vi "Add Correction.vi"(8 "error in (no error)":errorcluster, 9 "Assembly Type":string, 10 "XYZTheta":dbl[](array[numeric]), 11 "Carrier Tray in":refnum<class "Assembly Tray.lvclass">) -> (0 "error out":errorcluster, 2 "XYZTheta Out":dbl[](array[numeric]), 3 "Carrier Tray out":refnum<class "Assembly Tray.lvclass">)   [LabVIEW 2021, in "Assembly Tray.lvclass"]
uses:
  Assembly Tray.lvclass
  C:/Users/HEP/Documents/GitHub/Gantry/UCSB-Gantry-HEP-main/Classes/Workspace/Fixture.lvclass
  Fixture.lvclass/Fixture.ctl
  Read Fixture ID.vi
  Read Position.vi
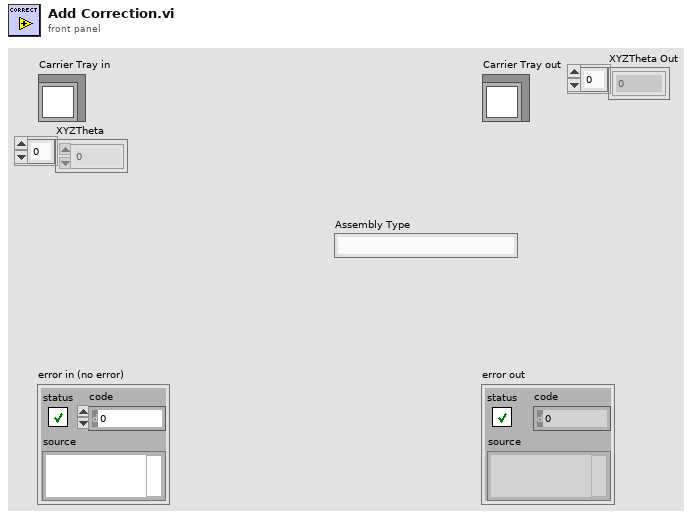
[diagram p1: front panel]
types:
  T1 = typedef "File Paths.ctl" = cluster{"Glue Pattern Folder":path, "Carrier Tray Folder":path, "Pick Up Tool Fixture Folder":path, "Components Folder":path, "Bellows Tool Offset.txt":path, "Pick Up Tool Offset.txt":path, "Dispense Tip Offset.txt":path, "Log Files":path, "Gantry Assembly Map.txt":path, "Syringe and offset map.txt":path, "Controllers Folder":path, "Local dbase config":path}
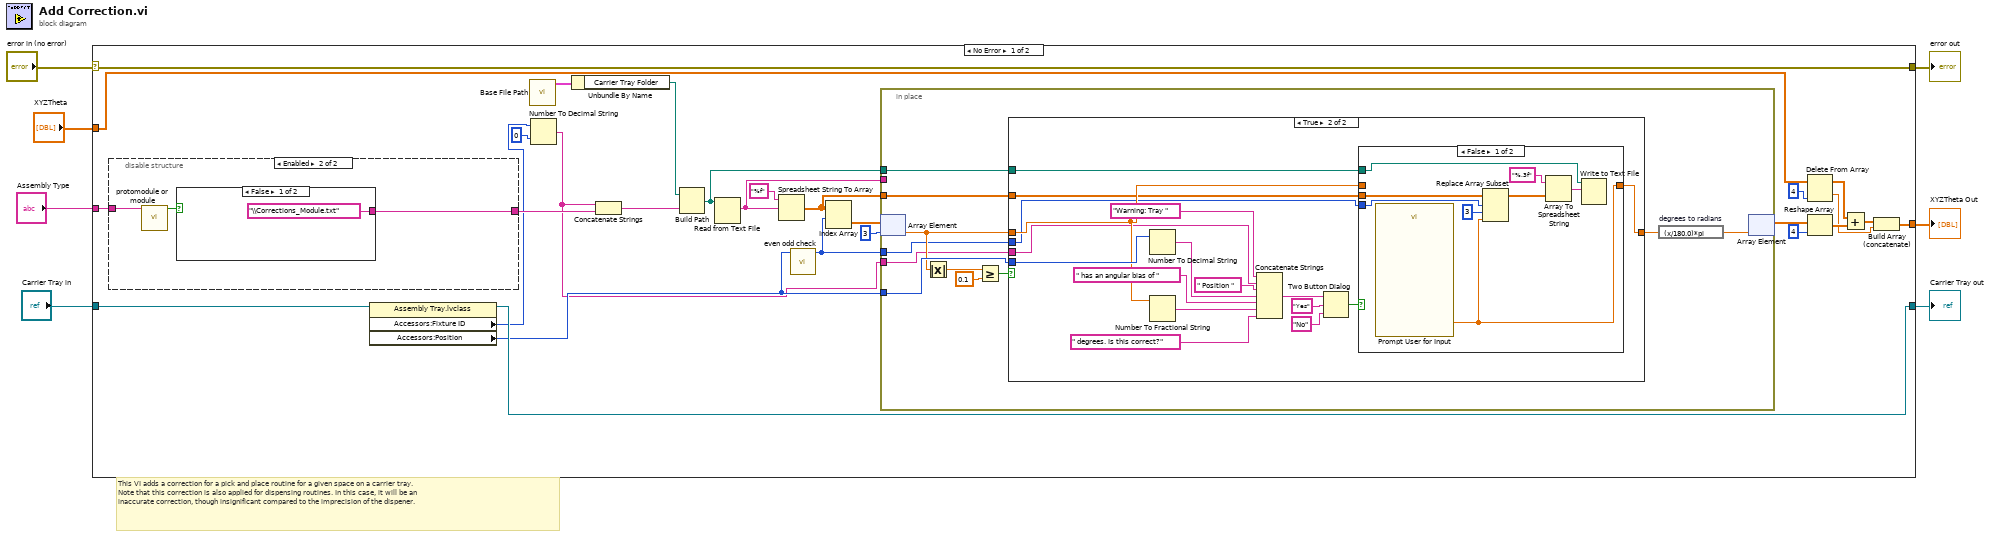
[diagram p0: block diagram]
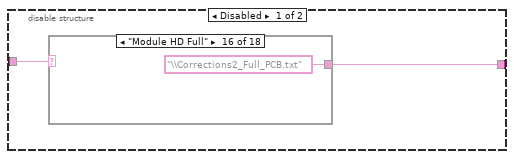
[diagram p4: hidden frame]
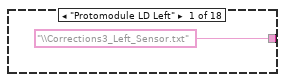
[diagram p5: hidden frame]
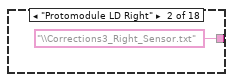
[diagram p6: hidden frame]
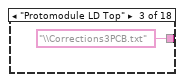
[diagram p7: hidden frame]
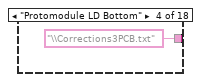
[diagram p8: hidden frame]
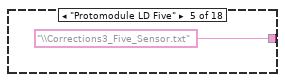
[diagram p9: hidden frame]
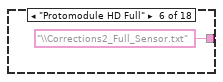
[diagram p10: hidden frame]
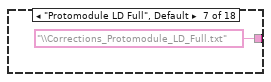
[diagram p11: hidden frame]
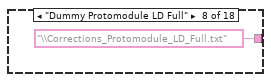
[diagram p12: hidden frame]
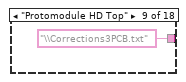
[diagram p13: hidden frame]
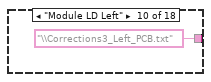
[diagram p14: hidden frame]
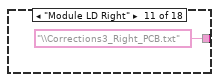
[diagram p15: hidden frame]
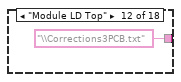
[diagram p16: hidden frame]
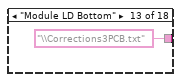
[diagram p17: hidden frame]
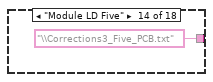
[diagram p18: hidden frame]
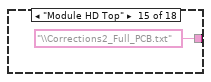
[diagram p19: hidden frame]
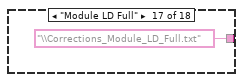
[diagram p20: hidden frame]
diagram:
  # "This VI adds a correction for a pick and place routine for a given space on a carrier tray.\nNote that this correction is also applied for dispensing routines. In this case, it will be an\ninaccurate correction, though insignificant compared to the imprecision of the dispener."
  n1 = case shown="No Error" "error in (no error)" {
    selector: "error in (no error)" -> [w35 w101]
    tunnel: [w35 w101] -> w6
    tunnel: [w25 w100] -> w4
    tunnel: "Carrier Tray in" -> [w26 w100]
    tunnel: "XYZTheta" -> [w22 w99]
    tunnel: [w17 w99] -> w2
    tunnel: "Assembly Type" -> [w23 _]
    frame No Error {
      n2 = disable-structure shown="Enabled" {
        disable-tunnel: [w75 w96] -> w31
        disable-tunnel: w23 -> [w74 w95]
        frame Disabled {
          n3 = case shown="\"Module HD Full\"" w74 {
            tunnel: ["\\Corrections3_Left_Sensor.txt" ("name or relative path") "\\Corrections3_Right_Sensor.txt" ("name or relative path") "\\Corrections3PCB.txt" ("name or relative path") "\\Corrections3PCB.txt" ("name or relative path") "\\Corrections3_Five_Sensor.txt" ("name or relative path") "\\Corrections2_Full_Sensor.txt" ("name or relative path") "\\Corrections_Protomodule_LD_Full.txt" ("name or relative path") "\\Corrections_Protomodule_LD_Full.txt" ("name or relative path") "\\Corrections3PCB.txt" ("name or relative path") "\\Corrections3_Left_PCB.txt" ("name or relative path") "\\Corrections3_Right_PCB.txt" ("name or relative path") "\\Corrections3PCB.txt" ("name or relative path") "\\Corrections3PCB.txt" ("name or relative path") "\\Corrections3_Five_PCB.txt" ("name or relative path") "\\Corrections2_Full_PCB.txt" ("name or relative path") "\\Corrections2_Full_PCB.txt" ("name or relative path") "\\Corrections_Module_LD_Full.txt" ("name or relative path") "\\Corrections_Module_LD_Full.txt" ("name or relative path")] -> w75
            frame "Protomodule LD Left" {
            }
            frame "Protomodule LD Right" {
            }
            frame "Protomodule LD Top" {
            }
            frame "Protomodule LD Bottom" {
            }
            frame "Protomodule LD Five" {
            }
            frame "Protomodule HD Full" {
            }
            frame "Protomodule LD Full", Default {
            }
            frame "Dummy Protomodule LD Full" {
            }
            frame "Protomodule HD Top" {
            }
            frame "Module LD Left" {
            }
            frame "Module LD Right" {
            }
            frame "Module LD Top" {
            }
            frame "Module LD Bottom" {
            }
            frame "Module LD Five" {
            }
            frame "Module HD Top" {
            }
            frame "Module HD Full" {
            }
            frame "Module LD Full" {
            }
            frame "Dummy Module LD Full" {
            }
          }
        }
        frame Enabled {
          n4 = call "protomodule or module.vi"("assembly type"=w95) -> ("protomodule? (T)"=w94:bool)  [unwired: 10 in]
          n5 = case shown="False" w94 {
            tunnel: ["\\Corrections_Module.txt" ("name or relative path") "\\Corrections_Protomodule.txt" ("name or relative path")] -> w96
            frame False {
            }
            frame True {
            }
          }
        }
      }
      n6 = property class="Assembly Tray.lvclass"(reference=w26) -> (reference out=w25:refnum<class "Assembly Tray.lvclass">, "Accessors:Fixture ID"=w24:i32, "Accessors:Position"=w14:i32)  [unwired: 1 in, 1 out]
      n7 = call "Base File Path.vi"() -> ("Paths Out"=w34:T1)  [unwired: 11 in]
      n8 = Number To Decimal String(number=w24, width (-)=i16 0) -> (decimal integer string=w13:string)
      n9 = Unbundle By Name(w34) -> ("Carrier Tray Folder"=w33:path)
      n10 = Concatenate Strings(w13, w31) -> (w30:string)
      n11 = Build Path(base path=w33, name or relative path=w30) -> (appended path=w11:path)
      n12 = Read from Text File(file (use dialog)=w11) -> (text=w15:string)  [unwired: 3 in, 3 out]
      n13 = Spreadsheet String To Array(format string="%f", spreadsheet string=w15) -> (array=w10:dbl[][])  [unwired: 2 in]
      n14 = call "even odd check.vi"("position"=w14) -> ("index"=w9:i32)  [unwired: 10 in]
      n15 = Index Array(array=w10, index (row)=w9) -> (element=w8:dbl[])  [unwired: 1 in]
      n16 = in-place {
        in-place-border: w15 -> [_]
        in-place-border: w14 -> [w41]
        in-place-border: w13 -> [w39]
        in-place-border: w11 -> [w38]
        in-place-border: w10 -> [w37]
        in-place-border: w9 -> [w36]
        n17 = in-place-array #1(w8, 3) -> (w40:dbl)
        n18 = Absolute Value(x=w40) -> (abs(x)=w45:dbl)
        n19 = Greater Or Equal?(x=w45, y=0.1) -> (x >= y?=w43:bool)
        n20 = case shown="True" w43 {
          tunnel: [w47 w56] -> w42
          tunnel: w41 -> [_ w61]
          tunnel: w40 -> [w47 w55]
          tunnel: w39 -> [_ w52]
          tunnel: w38 -> [_ w50]
          tunnel: w37 -> [_ w49]
          tunnel: w36 -> [_ w48]
          frame False {
          }
          frame True {
            n21 = Number To Decimal String(number=w61) -> (decimal integer string=w60:string)  [unwired: 1 in]
            n22 = Number To Fractional String(number=w55) -> (F-format string=w57:string)  [unwired: 3 in]
            n23 = Concatenate Strings("Warning: Tray " ("string"), w52, " Position " ("string"), w60, " has an angular bias of " ("string"), w57, " degrees. Is this correct?" ("string")) -> (w64:string)
            n24 = Two Button Dialog(message=w64, 1:"No" ("F button name (\"Cancel\")"), 2:"Yes" ("T button name (\"OK\")")) -> (T button?=w51:bool)
            n25 = case shown="False" w51 {
              tunnel: [w69 w73] -> w56
              tunnel: w55 -> [_ w73]
              tunnel: w50 -> [w70 _]
              tunnel: w49 -> [w68 _]
              tunnel: w48 -> [w67 _]
              frame False {
                n26 = call "Prompt User for Input"() -> ("angle_bias"=w69:dbl)  [unwired: 17 in, 2 out]
                n27 = Replace Array Subset(array=w68, new element=w69, index (row)=w67, index (col)=3 ("disabled index (col)")) -> (w65:dbl[][])
                n28 = Array To Spreadsheet String(array=w65, 3:"%.3f" ("format string")) -> (spreadsheet string=w72:string)  [unwired: 1 in]
                n29 = Write to Text File(file (use dialog)=w70, text=w72) -> ()  [unwired: 2 in, 3 out]
              }
              frame True {
              }
            }
          }
        }
        n30 = expression code="(x/180.0)*pi" "degrees to radians"(w42) -> (w46:dbl)
        n31 = in-place-array #1(w46) -> (w12:dbl[])  [unwired: 1 out]
      }
      n32 = Delete From Array(array=w22, index=4) -> (deleted portion=w18:dbl, array with subset deleted=w20:dbl[])  [unwired: 1 in]
      n33 = Reshape Array(w12, 4 ("dimension size")) -> (w27:dbl[])
      n34 = Add(x=w20, y=w27) -> (x+y=w19:dbl[])
      n35 = Build Array (concatenate)(w19, w18) -> (w17:dbl[])
    }
    frame Error {
    }
  }
  "error out" <- w6
  "Carrier Tray out" <- w4
  "XYZTheta Out" <- w2
